vi "PostTweet.vi"(8 "error in":errorcluster, 11 "Tweet":string) -> (0 "error out":errorcluster)   [LabVIEW 2014]
doc: "This example posts a text only tweet."
uses:
  <vilib>/LVH/i3 Twitter/SubVIs/Twitter Open - Embedded.vi
  <vilib>/LVH/i3 Twitter/Tweets/Post Tweet.vi
  <vilib>/LVH/i3 Twitter/i3-twitter.lvlib
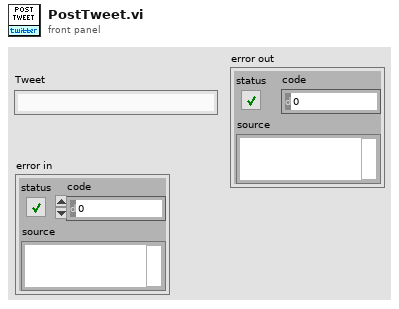
[diagram p1: front panel]
types:
  T1 = typedef "i3-twitter.lvlib/Twitter Handle.ctl" = cluster{"OAuth Credentials":T2, "since ID":string, "max ID":string, "Screen Name":string}
  T2 = typedef "i3-oauth.lvlib/OAuth Handle.ctl" = cluster{"Signature Method":T3, "Version":string, "Client":T4, "Access":T4}
  T3 = typedef "i3-oauth.lvlib/Signature Method.ctl" = enum16{"HMAC-MD5", "HMAC-SHA1", "HMAC-SHA224", "HMAC-SHA256", "HMAC-SHA384", "HMAC-SHA512"}
  T4 = typedef "i3-oauth.lvlib/Credentials.ctl" = cluster{"Token":string, "Secret":string}
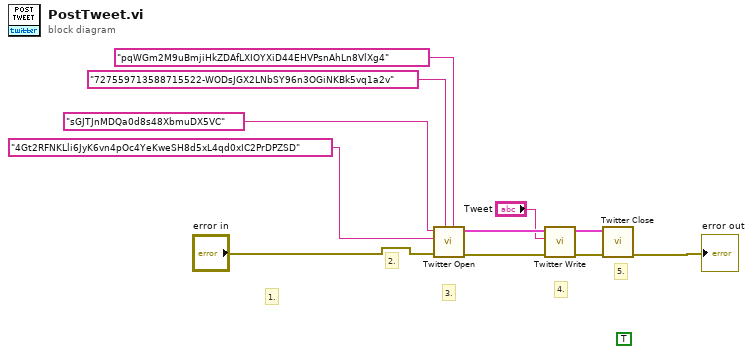
[diagram p0: block diagram]
diagram:
  (unwired) TRUE
  # "5."
  # "4."
  # "3."
  # "2."
  # "1."
  n1 = call-poly <vilib>:"Twitter Open.vi"("Access Secret"="pqWGm2M9uBmjiHkZDAfLXIOYXiD44EHVPsnAhLn8VlXg4", "Access Token"="727559713588715522-WODsJGX2LNbSY96n3OGiNKBk5vq1a2v", "error in"="error in", "Consumer Secret"="4Gt2RFNKLli6JyK6vn4pOc4YeKweSH8d5xL4qd0xIC2PrDPZSD", "Consumer Key"="sGJTJnMDQa0d8s48XbmuDX5VC") -> ("error out"=w9:errorcluster, "Twitter Handle Out"=w7:T1)  [unwired: 5 in]
  n2 = call-poly <vilib>:"Twitter Write.vi"("error in (no error)"=w9, "Tweet"="Tweet", "Twitter Handle In"=w7) -> ("error out"=w8:errorcluster, "Twitter Handle Out"=w6:T1)  [unwired: 7 in]
  n3 = call <vilib>:"Twitter Close.vi"("error in"=w8, "Twitter Handle In"=w6) -> ("error out"=→"error out":errorcluster)  [unwired: 9 in]
